vi "ATF-Error logger RT Storage.vi"(8 "error IO":errorcluster, 11 "?":T1) -> ()   [LabVIEW 2022 SP3]
uses:
  UI Message handler/Message Queue/All Message Queues.ctl
  UI Message handler/Message Queue/Message Cluster.ctl
  Controls/SeCrTs-Control error log.ctl
  c2162d36-98c9-4a30-90dd-13ba04aa1307.vi
  UI Message handler/Message Queue/Message Queue.lvlib
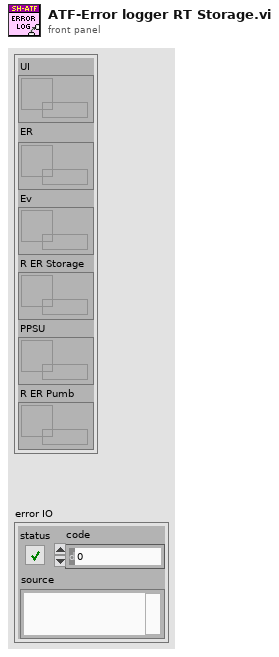
[diagram p1: front panel]
types:
  T1 = typedef "Message Queue.lvlib/All Message Queues.ctl" = cluster{"UI":refnum<queue>, "ER":refnum<queue>, "Ev":refnum<queue>, "R ER Storage":refnum<queue>, "PPSU":refnum<queue>, "R ER Pumb":refnum<queue>}
  T2 = typedef "SeCrTs-Control error log.ctl" = enum16{"Initialise", "Poll Event", "Logg Error", "Exit"}
  T3 = enum16{"open", "replace", "create", "open or create", "replace or create", "replace or create with confirmation"}
  T4 = typedef "SeCrTs-file folder ctl.ctl" = cluster{"Datalog path":path, "Configuration path":path, "Signal list path":path, "Sub vi's":path, "Authentication":path, "Sequence":path, "Event Log":path, "CS Error log":path, "RT Error Log":path}
  T5 = cluster{"Error Code":string, "Error Source":string}
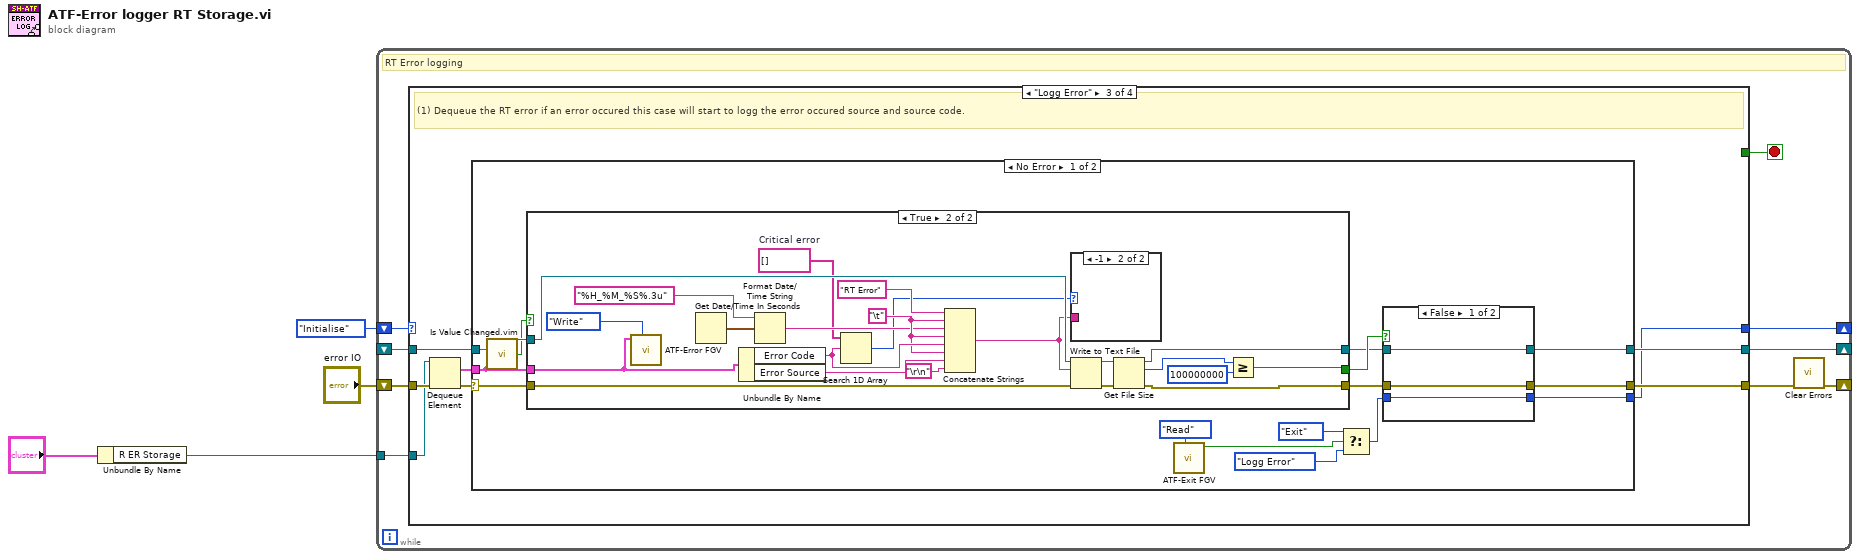
[diagram p0: block diagram]
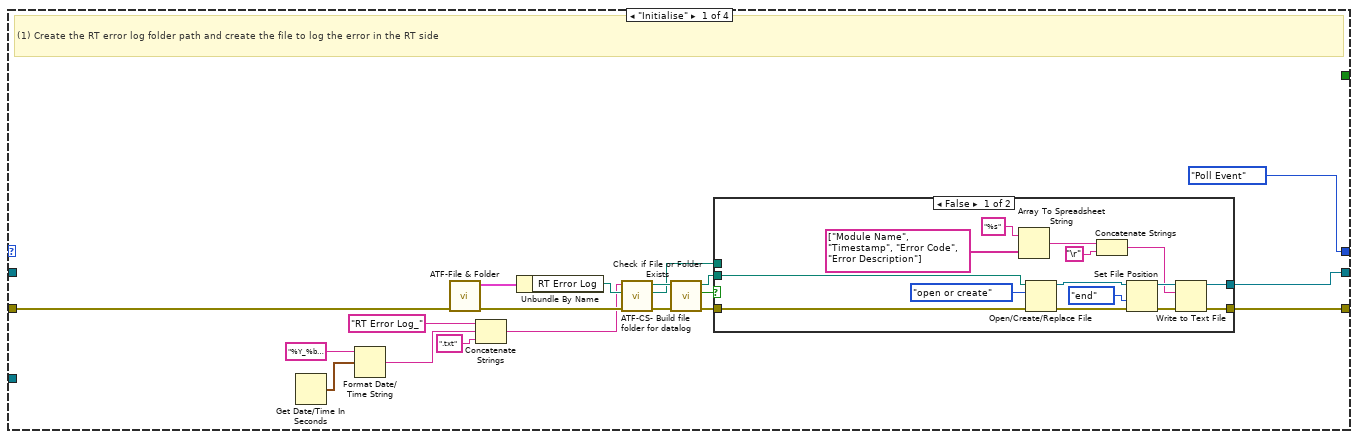
[diagram p2: hidden frame]
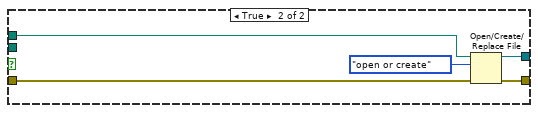
[diagram p3: hidden frame]
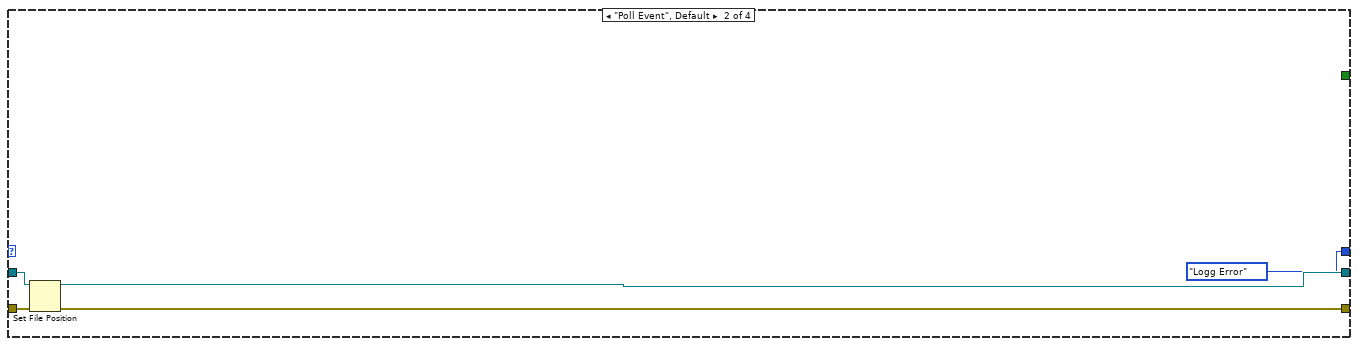
[diagram p4: hidden frame]
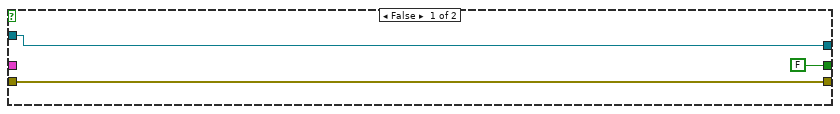
[diagram p5: hidden frame]
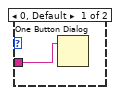
[diagram p6: hidden frame]
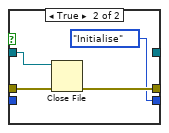
[diagram p7: hidden frame]
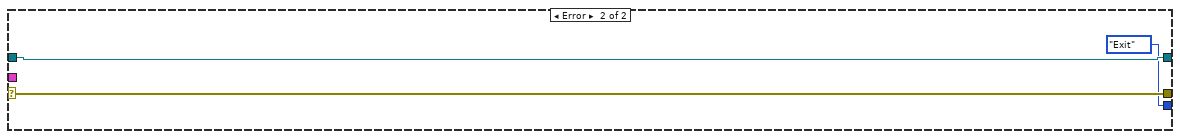
[diagram p8: hidden frame]
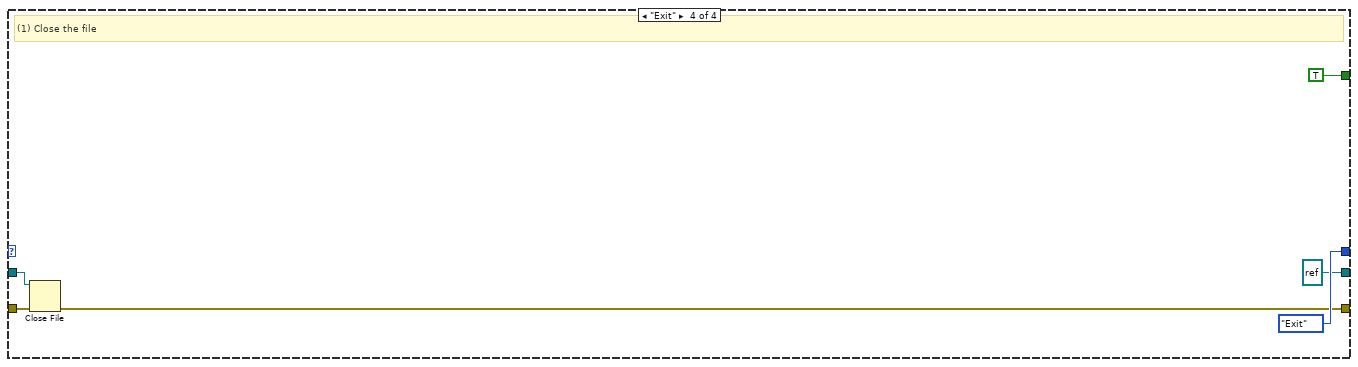
[diagram p9: hidden frame]
diagram:
  n1 = Unbundle By Name("?") -> ("R ER Storage"=w1:refnum<queue>)
  n2 = while {
    shift-right: [w12] -> _
    shift-left: SeCrTs-Control_error_log."Initialise" -> [w13]
    shift-right: [w11] -> _
    shift-left: _ -> [w10]
    shift-right: [w5] -> _
    shift-left: "error IO" -> [w9]
    tunnel: w1 -> [w6]
    stop <- w7 stop-if-true
    # "RT Error logging"
    n3 = case shown="\"Logg Error\"" w13 {
      tunnel: [SeCrTs-Control_error_log."Poll Event" SeCrTs-Control_error_log."Logg Error" w59 SeCrTs-Control_error_log."Exit"] -> w12
      tunnel: [w21 w56 w63 refnum<file> refnum ("refnum out")] -> w11
      tunnel: w10 -> [_ w57 w64 w120]
      tunnel: w9 -> [w18 w55 w61 w119]
      tunnel: [w19 w54 w62 w118] -> w8
      tunnel: [_ _ _ TRUE] -> w7
      tunnel: w6 -> [_ _ w58 _]
      frame "Initialise" {
        # "(1) Create the RT error log folder path and create the file to log the error in the RT side"
        n4 = Get Date/Time In Seconds() -> (seconds since 1Jan1904=w14:timestamp)
        n5 = Format Date/Time String(time format string (%c)="%Y_%b_%d_%Hh_%Mm_%Ssec", seconds (now)=w14) -> (date/time string=w27:string)  [unwired: 1 in]
        n6 = call "ATF-File & Folder.vi"("error in (no error)"=w18) -> ("error out"=w31:errorcluster, "File Output"=w32:T4)  [unwired: 9 in]
        n7 = Concatenate Strings("RT Error Log_" ("string"), w27, ".txt" ("string")) -> (w24:string)
        n8 = Unbundle By Name(w32) -> ("RT Error Log"=w30:path)
        n9 = call "ATF-CS- Build file folder for datalog.vi"("error in (no error)"=w31, "Base Path"=w30, "File Name"=w24) -> ("error out"=w28:errorcluster, "Result File path"=w16:path, "Result Folder path"=w29:path)  [unwired: 6 in]
        n10 = call <vilib>:"Check if File or Folder Exists.vi"("error in (no error)"=w28, "path"=w29) -> ("error out"=w20:errorcluster, "file or folder exists?"=w22:bool, "dup path"=w17:path)  [unwired: 7 in]
        n11 = case shown="False" w22 {
          tunnel: [w43 w51] -> w21
          tunnel: w20 -> [w46 w50]
          tunnel: [w42 w49] -> w19
          tunnel: w17 -> [w33 _]
          tunnel: w16 -> [_ w48]
          frame False {
            n12 = Array To Spreadsheet String(array=string[] ["Module Name", "Timestamp", "Error Code", "Error Description"], 3:"%s" ("format string")) -> (spreadsheet string=w37:string)  [unwired: 1 in]
            n13 = Open/Create/Replace File(file path (use dialog)=w33, error in=w46, operation (0:open)=T3."open or create") -> (refnum out=w45:refnum<file>, error out=w44:errorcluster)  [unwired: 3 in, 1 out]
            n14 = Concatenate Strings(w37, "\r") -> (w35:string)
            n15 = Set File Position(refnum=w45, from (0:start)=enum16{"start", "end", "current"}."end", error in=w44) -> (refnum out=w41:refnum<file>, error out=w40:errorcluster)  [unwired: 1 in]
            n16 = Write to Text File(file (use dialog)=w41, text=w35, error in=w40) -> (refnum out=w43:refnum<file>, error out=w42:errorcluster)  [unwired: 1 in, 1 out]
          }
          frame True {
            n17 = Open/Create/Replace File(file path (use dialog)=w48, error in=w50, operation (0:open)=T3."open or create") -> (refnum out=w51:refnum<file>, error out=w49:errorcluster)  [unwired: 3 in, 1 out]
          }
        }
      }
      frame "Poll Event", Default {
        n18 = Set File Position(refnum=w57, error in=w55) -> (refnum out=w56:refnum<file>, error out=w54:errorcluster)  [unwired: 2 in]
      }
      frame "Logg Error" {
        # "(1) Dequeue the RT error if an error occured this case will start to logg the error occured source and source code."
        n19 = Dequeue Element(queue=w58, error in (no error)=w61) -> (element=w65:T5, error out=w60:errorcluster)  [unwired: 1 in, 2 out]
        n20 = case shown="No Error" w60 {
          selector: w60 -> [w79 w116]
          tunnel: w65 -> [w68 _]
          tunnel: w64 -> [w80 w115]
          tunnel: [w74 w115] -> w63
          tunnel: [w76 w116] -> w62
          tunnel: [w73 SeCrTs-Control_error_log."Exit"] -> w59
          frame No Error {
            n21 = call "Is Value Changed.vim"("value"=w68) -> ("changed or first call?"=w66:bool)
            n22 = case shown="True" w66 {
              tunnel: w80 -> [w82 w105]
              tunnel: w79 -> [w81 w96]
              tunnel: [FALSE w91] -> w78
              tunnel: [w81 w90] -> w77
              tunnel: [w82 w89] -> w75
              tunnel: w68 -> [_ w84]
              frame False {
              }
              frame True {
                w98 = string[] []  # Critical error
                w101 = "\t"
                n23 = call "ATF-Error FGV.vi"("Enum"=enum16{"Read", "Write", "Clear"}."Write", "CS err"=w84) -> ()  [unwired: 9 in, 1 out]
                n24 = Get Date/Time In Seconds() -> (seconds since 1Jan1904=w86:timestamp)
                n25 = Unbundle By Name(w84) -> ("Error Code"=w104:string, "Error Source"=w103:string)
                n26 = Format Date/Time String(time format string (%c)="%H_%M_%S%.3u", seconds (now)=w86) -> (date/time string=w100:string)  [unwired: 1 in]
                n27 = Search 1D Array(1D array=w98, element=w104) -> (index of element=w97:i32)  [unwired: 1 in]
                n28 = Concatenate Strings("RT Error" ("string"), w101, w100, w101, w104, w101, w103, "\r\n") -> (w88:string)
                n29 = case shown="-1" w97 {
                  tunnel: w88 -> [w106 _]
                  frame 0, Default {
                    n30 = One Button Dialog(message=w106) -> ()  [unwired: 1 in, 1 out]
                  }
                  frame -1 {
                  }
                }
                n31 = Write to Text File(file (use dialog)=w105, text=w88, error in=w96) -> (refnum out=w94:refnum<file>, error out=w95:errorcluster)  [unwired: 1 in, 1 out]
                n32 = Get File Size(file=w94, error in=w95) -> (refnum out=w89:refnum<file>, size (in bytes)=w93:i64, 0:w90:errorcluster)
                n33 = Greater Or Equal?(x=w93, y=i64 100000000) -> (x >= y?=w91:bool)
              }
            }
            n34 = call "ATF-Exit FGV.vi"("Enum"=enum16{"Init", "Read", "Write"}."Read") -> ("Exit R"=w70:bool)  [unwired: 9 in, 1 out]
            n35 = Select(t=SeCrTs-Control_error_log."Exit", s=w70, f=SeCrTs-Control_error_log."Logg Error") -> (s? t:f=w72:T2)
            n36 = case shown="False" w78 {
              tunnel: w77 -> [w109 w111]
              tunnel: [w109 w112] -> w76
              tunnel: w75 -> [w108 w113]
              tunnel: [w108 _] -> w74
              tunnel: [w107 SeCrTs-Control_error_log."Initialise"] -> w73
              tunnel: w72 -> [w107 _]
              frame False {
              }
              frame True {
                n37 = Close File(refnum=w113, error in=w111) -> (error out=w112:errorcluster)  [unwired: 1 out]
              }
            }
          }
          frame Error {
          }
        }
      }
      frame "Exit" {
        # "(1) Close the file"
        n38 = Close File(refnum=w120, error in=w119) -> (error out=w118:errorcluster)  [unwired: 1 out]
      }
    }
    n39 = call <vilib>:"Clear Errors.vi"("error in (no error)"=w8) -> ("error out"=w5:errorcluster)  [unwired: 5 in, 1 out]
  }
